vi "protocol.vi"() -> ()   [LabVIEW 2016]
uses:
  <vilib>/Instr/_visa.llb/VISA Configure Serial Port (Instr).vi
panel:
  in  "stop":bool
  out "return count":u32
  out "error out":errorcluster
  in  "termination char\n(0xA = '\\n' = LF)":u8=10 format="%.0x"
  in  "VISA resource name":refnum<visa-resource-name>
  in  "Serial Settings":T1={"baud rate"=9600, "data bits"=8, "parity"=enum."None", "stop bits"=10, "flow control"=0} {"flow control" items=["None"=0, "XON/XOFF"=1, "RTS/CTS"=2, "DTR/DSR"=4]; "stop bits" items=["1.0"=10, "1.5"=15, "2.0"=20]; "data bits" min=5 max=8 step=1; "baud rate" items=["75"=75, "110"=110, "134"=134, "150"=150, "300"=300, "600"=600, "1200"=1200, "1800"=1800, "2400"=2400, "4800"=4800, "7200"=7200, "9600"=9600, "14400"=14400, "19200"=19200, "28800"=28800, "38400"=38400, "56000"=56000, "57600"=57600, "115200"=115200, "128000"=128000, "230400"=230400]}
  in  "vel radial":i16
  in  "vel normal":i16
  in  "vel rotation":i16
  in  "pos 3":i16=3468
  out "unsigned byte array 3":u8[](array[numeric])
  in  "pos 2":i16=3468
  out "unsigned byte array 2":u8[](array[numeric])
  in  "pos 1":i16=3468
  out "unsigned byte array":u8[](array[numeric])
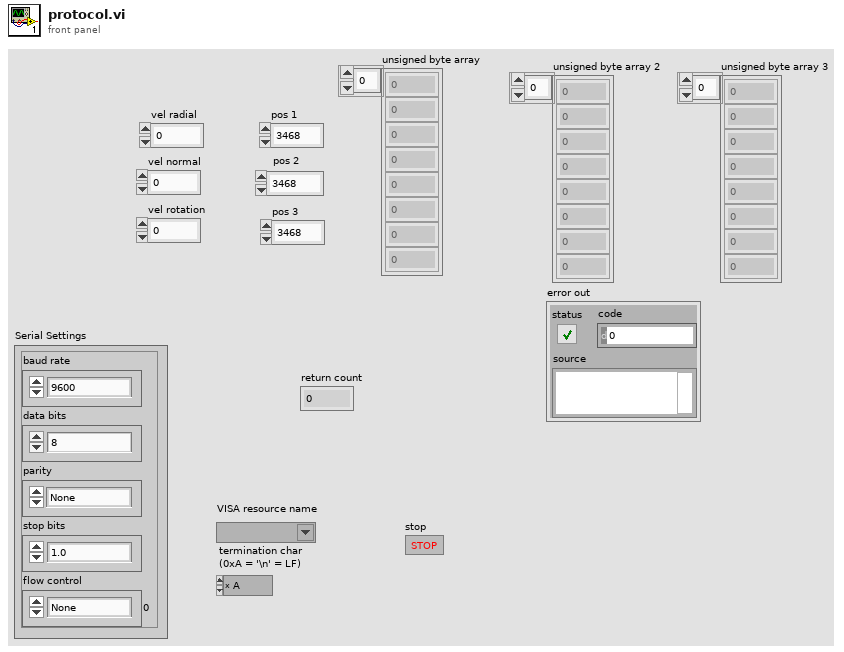
[diagram p1: front panel]
types:
  T1 = cluster{"baud rate":u32, "data bits":u16, "parity":enum16{"None", "Odd", "Even", "Mark", "Space"}, "stop bits":u16, "flow control":u16}
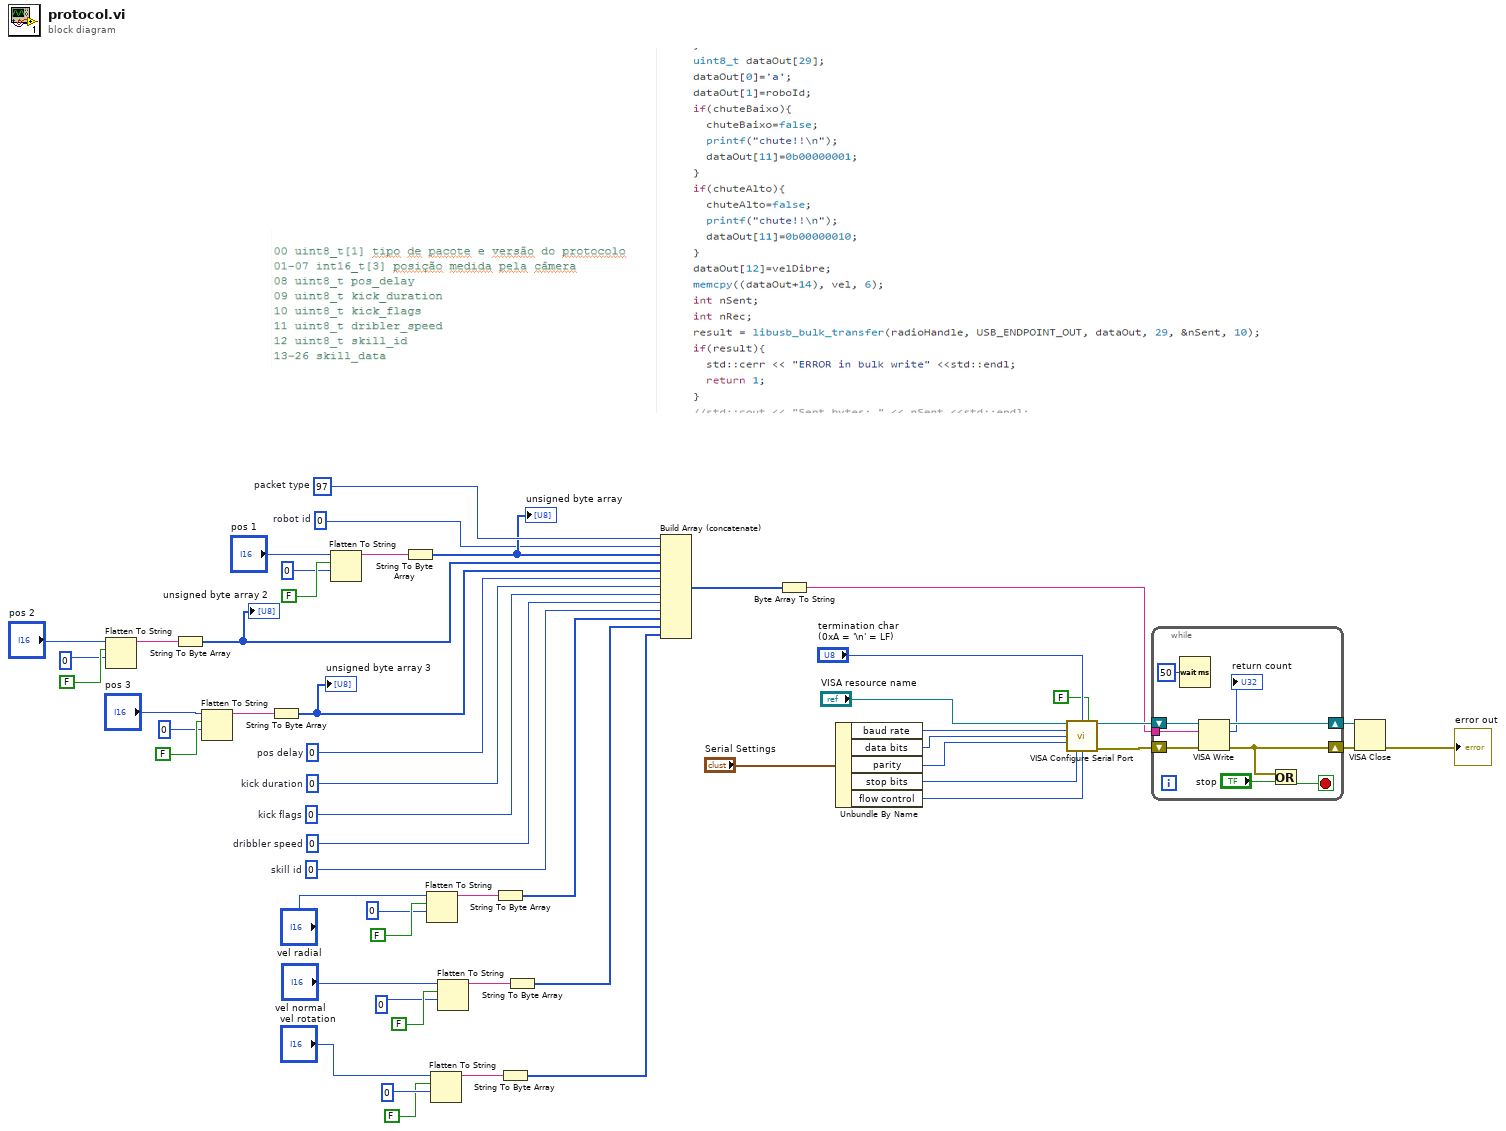
[diagram p0: block diagram]
diagram:
  w23 = u8 0  # skill id
  w52 = u8 0  # dribbler speed
  w18 = u8 0  # kick flags
  w24 = u8 0  # kick duration
  w25 = u8 0  # pos delay
  w20 = u8 0  # robot id
  w53 = u8 97  # packet type
  n1 = Flatten To String(anything="pos 2", prepend array or string size? (T)=FALSE, byte order (0:big-endian, network order)=u16 0) -> (data string=w44:string)  [unwired: 1 in, 2 out]
  n2 = String To Byte Array(string=w44) -> (unsigned byte array=w19:u8[])
  "unsigned byte array 2" <- w19
  n3 = Flatten To String(anything="pos 3", prepend array or string size? (T)=FALSE, byte order (0:big-endian, network order)=u16 0) -> (data string=w40:string)  [unwired: 1 in, 2 out]
  n4 = String To Byte Array(string=w40) -> (unsigned byte array=w38:u8[])
  "unsigned byte array 3" <- w38
  n5 = Flatten To String(anything="pos 1", prepend array or string size? (T)=FALSE, byte order (0:big-endian, network order)=u16 0) -> (data string=w49:string)  [unwired: 1 in, 2 out]
  n6 = String To Byte Array(string=w49) -> (unsigned byte array=w48:u8[])
  "unsigned byte array" <- w48
  n7 = Flatten To String(anything="vel radial", prepend array or string size? (T)=FALSE, byte order (0:big-endian, network order)=u16 0) -> (data string=w35:string)  [unwired: 1 in, 2 out]
  n8 = Flatten To String(anything="vel rotation", prepend array or string size? (T)=FALSE, byte order (0:big-endian, network order)=u16 0) -> (data string=w29:string)  [unwired: 1 in, 2 out]
  n9 = Flatten To String(anything="vel normal", prepend array or string size? (T)=FALSE, byte order (0:big-endian, network order)=u16 0) -> (data string=w30:string)  [unwired: 1 in, 2 out]
  n10 = String To Byte Array(string=w35) -> (unsigned byte array=w33:u8[])
  n11 = String To Byte Array(string=w29) -> (unsigned byte array=w26:u8[])
  n12 = String To Byte Array(string=w30) -> (unsigned byte array=w27:u8[])
  n13 = Build Array (concatenate)(w53, w20, w48, w19, w38, w25, w24, w18, w52, w23, w33, w27, w26) -> (w2:u8[])
  n14 = Byte Array To String(unsigned byte array=w2) -> (string=w1:string)
  n15 = Unbundle By Name("Serial Settings") -> ("baud rate"=w15:u32, "data bits"=w14:u16, "parity"=w13:enum16{"None", "Odd", "Even", "Mark", "Space"}, "stop bits"=w12:u16, "flow control"=w11:u16)
  n16 = call-poly "VISA Configure Serial Port"("VISA resource name"="VISA resource name", "termination char\n(0xA = '\\n' = LF)"="termination char\n(0xA = '\\n' = LF)", "Enable Termination\nChar (T)"=FALSE ("Enable Termination\nChar (T)"), "baud rate (9600)"=w15, "data bits (8)"=w14, "parity (0:none)"=w13, "stop bits (10: 1 bit)"=w12, "flow control (0:none)"=w11) -> ("VISA resource name out"=w7:refnum<visa-resource-name>, "error out"=w5:errorcluster)  [unwired: 6 in]
  n17 = while {
    tunnel: w1 -> [w59]
    shift-right: [w61] -> w6
    shift-left: w7 -> [w62]
    shift-right: [w55] -> w4
    shift-left: w5 -> [w60]
    stop <- w56 stop-if-true
    n18 = Wait (ms)(milliseconds to wait=u32 50) -> ()  [unwired: 1 out]
    n19 = VISA Write(VISA resource name=w62, write buffer=w59, error in (no error)=w60) -> (VISA resource name out=w61:refnum<visa-resource-name>, return count=→"return count":u32, error out=w55:errorcluster)
    n20 = Or(x=w55, y="stop") -> (x .or. y?=w56:bool)
  }
  n21 = VISA Close(VISA resource name=w6, error in (no error)=w4) -> (error out=→"error out":errorcluster)
